vi "lockinmodificado.vi"() -> ()   [LabVIEW 2016]
panel:
  in  "Campo inicial":dbl
  in  "Delay Time (s)":dbl=30.0
  out "Girar 4":bool
  out "Girar 3":bool
  out "Girar 2":bool
  out "Midiendo":bool
  out "Girar":bool
  in  "Incremento":dbl
  out "error out":errorcluster
  in  "Nombre (guardar como .txt)":path
  out "Campo actual":dbl
  out "L/M":cluster{"array":dbl[], "array":dbl[]}(graph)
  out "Multimetro":cluster{"array":dbl[], "array":dbl[]}(graph)
  out "Lock_In":cluster{"array":dbl[], "array":dbl[]}(graph)
  in  "Campo Final":dbl
  in  "Lecturas":i32=1
  in  "Delay(ms)":u32
  in  "Tipo":u16(ring)=1 items=["LockIn", "LockIn-DMM"]
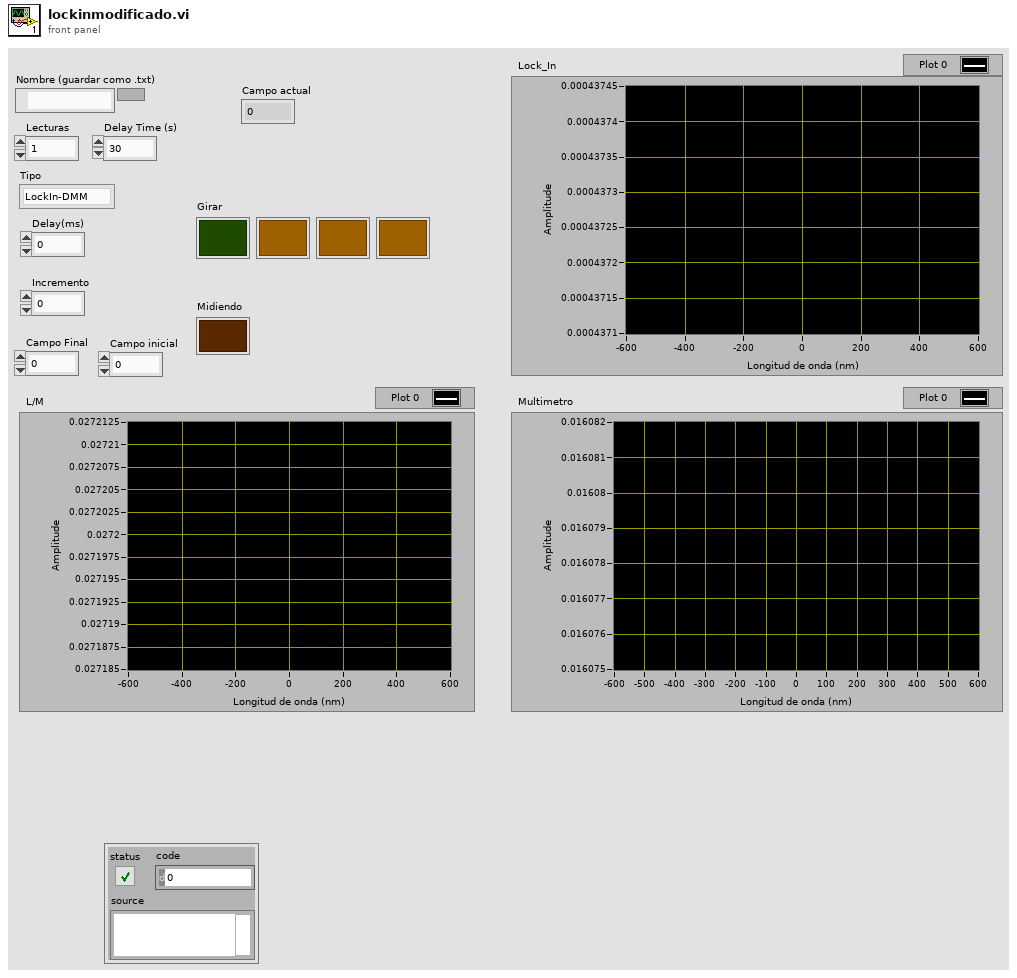
[diagram p1: front panel]
types:
  T1 = enum16{"open", "replace", "create", "open or create", "replace or create", "replace or create with confirmation"}
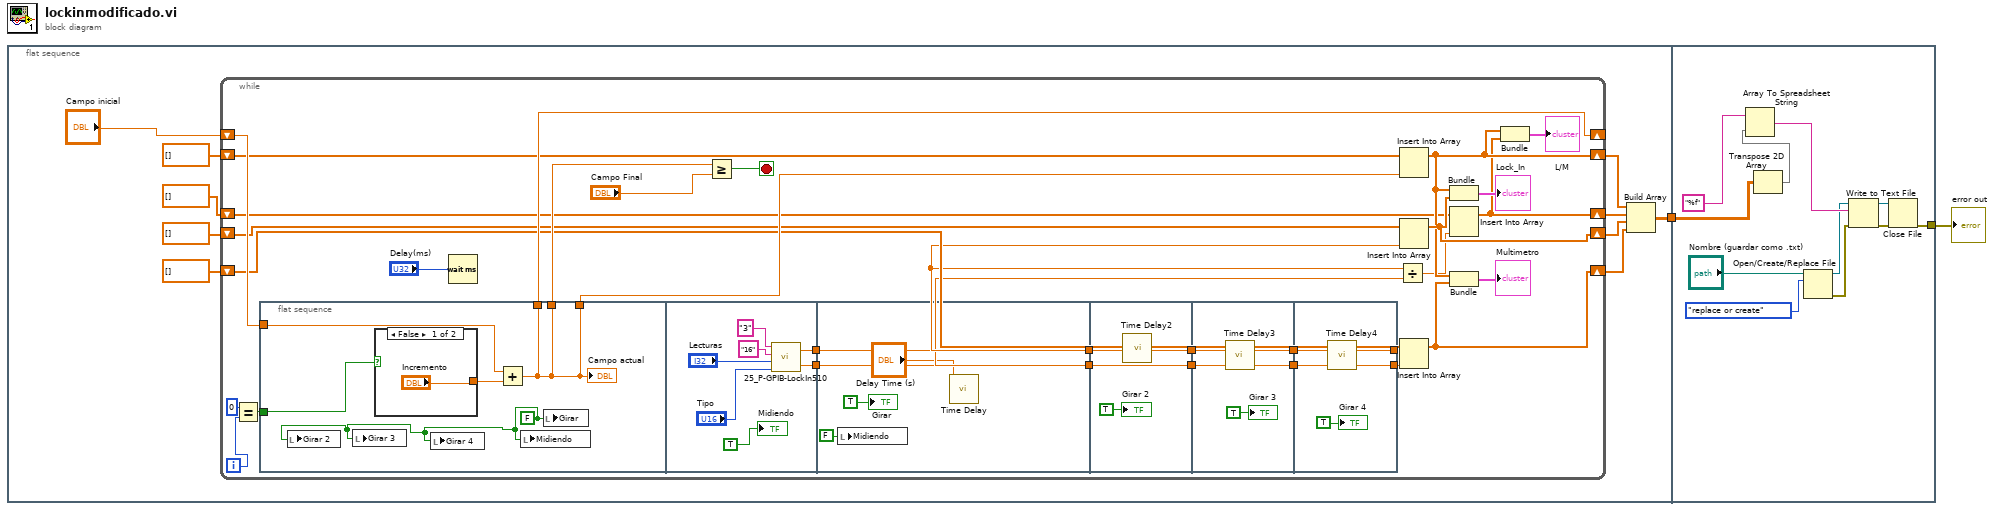
[diagram p0: block diagram]
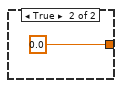
[diagram p2: hidden frame]
diagram:
  n1 = flat-sequence {
    tunnel: [w4] -> w2
    tunnel: w2 -> [w74]
    tunnel: [w75] -> w1
    frame #0 {
      n2 = while {
        shift-right: [w39] -> _
        shift-left: "Campo inicial" -> [w40]
        shift-right: [w32] -> w8
        shift-left: dbl[] [] ("array") -> [w37]
        shift-right: [w34] -> w6
        shift-left: dbl[] [] ("array") -> [w36]
        shift-right: [w31] -> w5
        shift-left: dbl[] [] ("array") -> [w35]
        shift-right: [w25] -> w7
        shift-left: dbl[] [] ("array") -> [w26]
        i -> [w23]
        stop <- w41 stop-if-true
        n3 = Equal?(x=0, y=w23) -> (x = y?=w21:bool)
        n4 = flat-sequence {
          tunnel: [w47] -> w43
          tunnel: w40 -> [w49]
          tunnel: [w47] -> w39
          tunnel: [w47] -> w38
          tunnel: w21 -> [w46]
          tunnel: [w54] -> w20
          tunnel: [w53] -> w19
          tunnel: w20 -> [w63]
          tunnel: w19 -> [w62]
          tunnel: [w63] -> w18
          tunnel: [w62] -> w17
          tunnel: w18 -> [w66]
          tunnel: w17 -> [w65]
          tunnel: [w66] -> w16
          tunnel: [w65] -> w15
          tunnel: w16 -> [w69]
          tunnel: w15 -> [w68]
          tunnel: [w69] -> w14
          tunnel: [w68] -> w13
          tunnel: [w71] -> w28
          tunnel: [w72] -> w29
          tunnel: w14 -> [w72]
          tunnel: w13 -> [w71]
          frame #0 {
            w45 = FALSE ("Girar")
            n5 = local write "Girar 2"(w45) -> ()
            n6 = local write "Girar 3"(w45) -> ()
            n7 = case shown="False" w46 {
              tunnel: ["Incremento" 0.0 ("Incremento")] -> w48
              frame False {
              }
              frame True {
              }
            }
            n8 = local write "Girar 4"(w45) -> ()
            n9 = Add(x=w49, y=w48) -> (x+y=w47:dbl)
            "Campo actual" <- w47
            n10 = local write "Midiendo"(w45) -> ()
            n11 = local write "Girar"(w45) -> ()
          }
          frame #1 {
            n12 = call "25_P-GPIB-LockIn510.vi"("Tipo"="Tipo", "Lecturas"="Lecturas", "P-DMM"="16", "P-LockIn"="3") -> ("DMM"=w53:dbl, "LockIn"=w54:dbl)
            "Midiendo" <- TRUE
          }
          frame #2 {
            n13 = local write "Midiendo"(FALSE ("Midiendo")) -> ()
            n14 = call "Time Delay"("Delay Time (s)"="Delay Time (s)") -> ()  [unwired: 10 in, 1 out]
            "Girar" <- TRUE ("Girar")
          }
          frame #3 {
            n15 = call "Time Delay2"() -> ()  [unwired: 11 in, 1 out]
            "Girar 2" <- TRUE ("Girar 2")
          }
          frame #4 {
            n16 = call "Time Delay3"() -> ()  [unwired: 11 in, 1 out]
            "Girar 3" <- TRUE ("Girar 3")
          }
          frame #5 {
            n17 = call "Time Delay4"() -> ()  [unwired: 11 in, 1 out]
            "Girar 4" <- TRUE ("Girar 4")
          }
        }
        n18 = Wait (ms)(milliseconds to wait="Delay(ms)") -> ()  [unwired: 1 out]
        n19 = Greater Or Equal?(x=w43, y="Campo Final") -> (x >= y?=w41:bool)
        n20 = Divide(x=w29, y=w28) -> (x/y=w27:dbl)
        n21 = Insert Into Array(array=w37, new element=w38) -> (w32:dbl[])  [unwired: 1 in]
        n22 = Insert Into Array(array=w36, new element=w29) -> (w34:dbl[])  [unwired: 1 in]
        n23 = Insert Into Array(array=w35, new element=w28) -> (w31:dbl[])  [unwired: 1 in]
        n24 = Bundle("array"=w32, "array"=w34) -> (→"Lock_In":cluster{"array":dbl[], "array":dbl[]})  [unwired: 1 in]
        n25 = Insert Into Array(array=w26, new element=w27) -> (w25:dbl[])  [unwired: 1 in]
        n26 = Bundle("array"=w32, "array"=w31) -> (→"Multimetro":cluster{"array":dbl[], "array":dbl[]})  [unwired: 1 in]
        n27 = Bundle("array"=w32, "array"=w25) -> (→"L/M":cluster{"array":dbl[], "array":dbl[]})  [unwired: 1 in]
      }
      n28 = Build Array(w8, w7, w6, w5) -> (w4:dbl[][])
    }
    frame #1 {
      n29 = Transpose 2D Array(2D array=w74) -> (transposed array=w73:dbl[][])
      n30 = Array To Spreadsheet String(array=w73, 3:"%f" ("format string")) -> (spreadsheet string=w82:string)  [unwired: 1 in]
      n31 = Open/Create/Replace File(file path (use dialog)="Nombre (guardar como .txt)", operation (0:open)=T1."replace or create") -> (refnum out=w81:refnum<file>, error out=w80:errorcluster)  [unwired: 4 in, 1 out]
      n32 = Write to Text File(file (use dialog)=w81, text=w82, error in=w80) -> (refnum out=w78:refnum<file>, error out=w79:errorcluster)  [unwired: 1 in, 1 out]
      n33 = Close File(refnum=w78, error in=w79) -> (error out=w75:errorcluster)  [unwired: 1 out]
    }
  }
  "error out" <- w1
